vi "Sending Params.vi"(10 "Sending Params":T1, 11 "Interval (100)":i32=100 min=1 max=10000 step=1) -> (1 "params out":string, 2 "which params":string, 3 "params array out":string[](array[string]))   [LabVIEW 2021, in "STAV lib.lvlib"]
uses:
  STAV lib.lvlib
  Sending Params.ctl
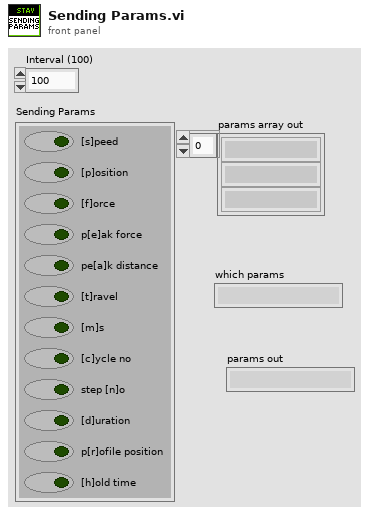
[diagram p1: front panel]
types:
  T1 = typedef "STAV lib.lvlib/Sending Params.ctl" = cluster{"[s]peed":bool, "[p]osition":bool, "[f]orce":bool, "p[e]ak force":bool, "pe[a]k distance":bool, "[t]ravel":bool, "[m]s":bool, "[c]ycle no":bool, "step [n]o":bool, "[d]uration":bool, "p[r]ofile position":bool, "[h]old time":bool}
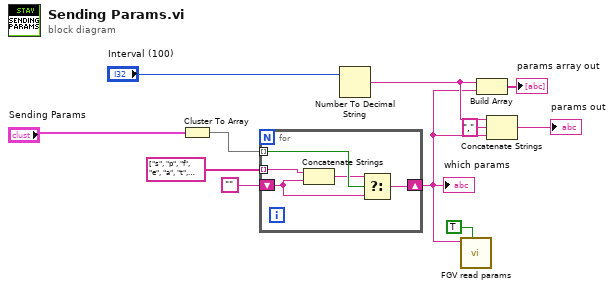
[diagram p0: block diagram]
diagram:
  n1 = Cluster To Array(cluster="Sending Params") -> (array=w9:bool[])
  n2 = for {
    tunnel: string[] ["s", "p", "f", "e", "a", "t", "m", "c", "n", "d", "r", "h"] -> [w12] mode=indexing
    tunnel: w9 -> [w16] mode=indexing
    shift-right: [w15] -> w2
    shift-left: "" -> [w13]
    n3 = Concatenate Strings(w12, w13) -> (w14:string)
    n4 = Select(t=w14, s=w16, f=w13) -> (s? t:f=w15:string)
  }
  "which params" <- w2
  n5 = Number To Decimal String(number="Interval (100)") -> (decimal integer string=w4:string)  [unwired: 1 in]
  n6 = call "FGV read params.vi"("Write (F)"=TRUE, "params in"=w2) -> ()  [unwired: 9 in, 1 out]
  n7 = Build Array(w4, w2) -> (→"params array out":string[])
  n8 = Concatenate Strings(w4, "," ("string"), w2) -> (→"params out":string)
